vi "MLX Prog NVRAM.vi"(7 "nad":u8, 9 "nvramFileName":string, 10 "LINChannel":u8, 11 "DeviceHandle":i32) -> (3 "function return":i32)   [LabVIEW 2010, in "mlx_programer.lvlib"]
doc: "int MLX_ProgNVRAM(int DeviceHandle, unsigned char LINChannel,const char* nvramFileName, unsigned char nad);"
uses:
  mlx_programer.lvlib
  USB2XXX/trunk/USB2XXX/USB2XXX/vs2010/Release/USB2XXX.dll
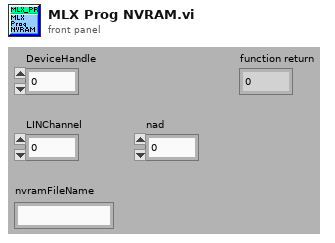
[diagram p1: front panel]
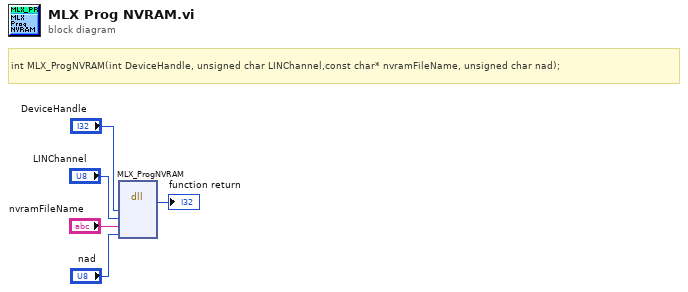
[diagram p0: block diagram]
diagram:
  # "int MLX_ProgNVRAM(int DeviceHandle, unsigned char LINChannel,const char* nvramFileName, unsigned char nad);"
  n1 = dll-call lib="E:/Projects/USB2XXX/trunk/USB2XXX/USB2XXX/vs2010/Release/USB2XXX.*" fn="MLX_ProgNVRAM"("DeviceHandle"="DeviceHandle", "LINChannel"="LINChannel", "nvramFileName"="nvramFileName", "nad"="nad") -> (→"function return":i32)  [unwired: 7 in, 2 out]
